vi "AutoIntake.vi"   [LabVIEW 2014]
uses:
  Robot Global Data.vi
types:
  T1 = typedef "WPI_DigitalInputDevRef.ctl" = cluster{"DevStatus":errorcluster, "DIO Channel":T2, "Controller":T3}
  T2 = typedef "FPGA_DIOChannel.ctl" = enum8{"DIO 0", "DIO 1", "DIO 2", "DIO 3", "DIO 4", "DIO 5", "DIO 6", "DIO 7", "DIO 8", "DIO 9", "DIO MXP 0", "DIO MXP 1", "DIO MXP 2", "DIO MXP 3", "DIO MXP 4", "DIO MXP 5", "DIO MXP 6", "DIO MXP 7", "DIO MXP 8", "DIO MXP 9", "DIO MXP 10", "DIO MXP 11", "DIO MXP 12", "DIO MXP 13", "DIO MXP 14", "DIO MXP 15", "Invalid"}
  T3 = typedef "FPGA_TypedefDigitalModule.ctl" = enum16{"Controller 1"}
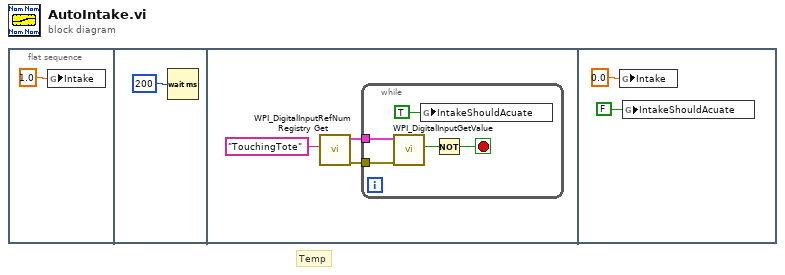
[diagram p0: block diagram]
diagram:
  # "Temp"
  n1 = flat-sequence {
    frame #0 {
      n2 = global write "Robot Global Data.vi" "Intake"(1.0) -> ()
    }
    frame #1 {
      n3 = Wait (ms)(milliseconds to wait=u32 200) -> ()  [unwired: 1 out]
    }
    frame #2 {
      n4 = call <vilib>:"WPI_DigitalInputRefNum Registry Get.vi"("refnum name"="TouchingTote") -> ("error out"=w3:errorcluster, "DigitalInputDevRef"=w4:T1)  [unwired: 9 in]
      n5 = while {
        tunnel: w4 -> [w10]
        tunnel: w3 -> [w9]
        stop <- w8 stop-if-true
        n6 = call <vilib>:"WPI_DigitalInputGetValue.vi"("error in (no error)"=w9, "DigitalInputDevRef"=w10) -> ("Value"=w7:bool)  [unwired: 7 in, 2 out]
        n7 = global write "Robot Global Data.vi" "IntakeShouldAcuate"(TRUE) -> ()
        n8 = Not(x=w7) -> (.not. x?=w8:bool)
      }
    }
    frame #3 {
      n9 = global write "Robot Global Data.vi" "Intake"(0.0) -> ()
      n10 = global write "Robot Global Data.vi" "IntakeShouldAcuate"(FALSE) -> ()
    }
  }
